vi "Vision Research Phantom Series VI Tree.vi"   [LabVIEW 2013, in "VRI.lvlib"]
doc: "This is the instrument driver for the Dresser DXD Series Precision Digital Pressure Transducer. The VI Tree displays all the user-callable VIs of the instrument driver in an organized table. Look at the \"Getting Started\" VI's to get an idea of how to use this driver in your application."
uses:
  VRI.lvlib
panel:
  # "Vision Research\nPhantom Series\nCamera\nLabVIEW Driver"
  # "SEE DIAGRAM\nFOR VI TREE."
  # "Version 3.0.770.0"
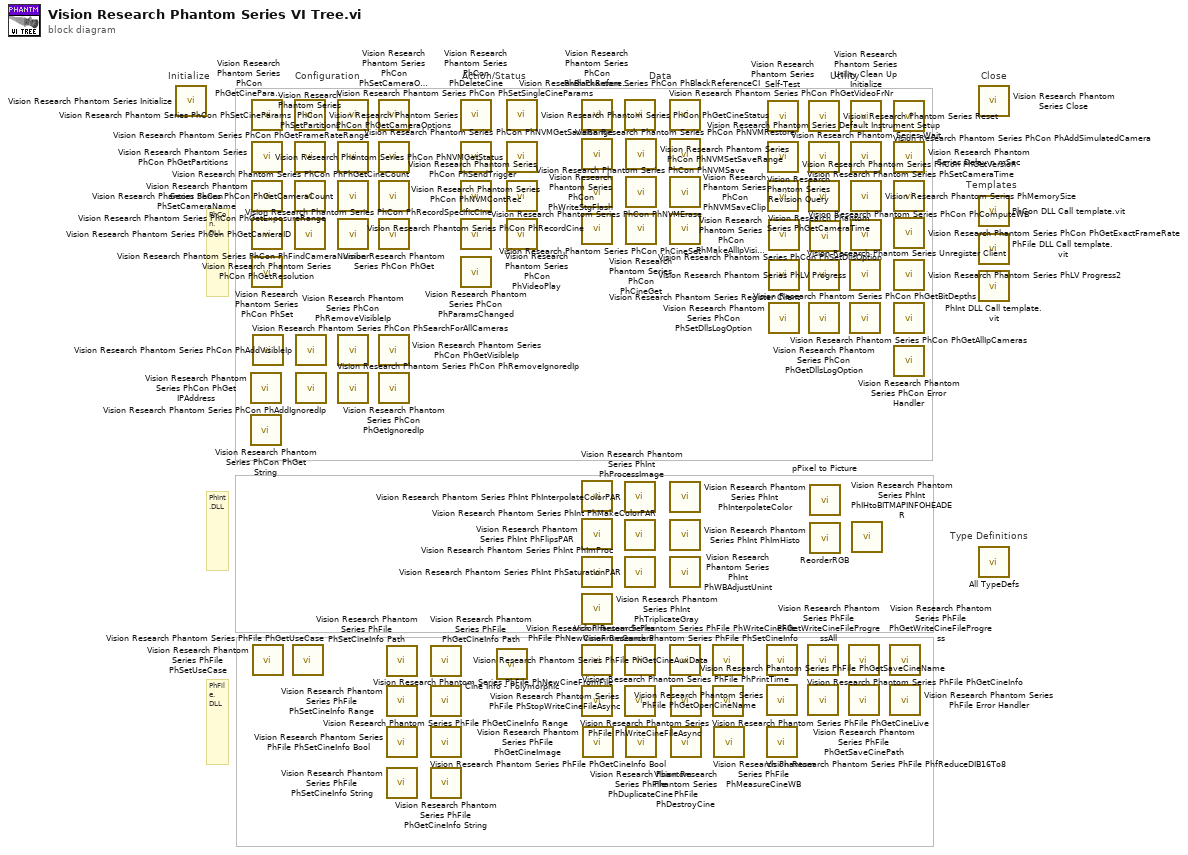
[diagram p0: block diagram]
diagram:
  # "Type Definitions"
  # "PhFile.DLL"
  # "PhInt.DLL"
  # "PhCon.DLL"
  # "Templates"
  # "Configuration"
  # "Utility"
  # "Data"
  # "Action/Status"
  # "Close"
  # "Initialize"
  n1 = call "Vision Research Phantom Series Initialize.vi"() -> ()  [unwired: 5 in, 15 out]
  n2 = call "Vision Research Phantom Series PhCon PhGet IPAddress.vi"() -> ()  [unwired: 17 in, 3 out]
  n3 = call "Vision Research Phantom Series PhCon PhGet String.vi"() -> ()  [unwired: 17 in, 3 out]
  n4 = call "Vision Research Phantom Series PhCon PhGetCineParams.vi"() -> ()  [unwired: 3 in, 17 out]
  n5 = call "Vision Research Phantom Series PhCon PhGetPartitions.vi"() -> ()  [unwired: 3 in, 17 out]
  n6 = call "Vision Research Phantom Series PhCon PhSetCameraName.vi"() -> ()  [unwired: 3 in, 17 out]
  n7 = call "Vision Research Phantom Series PhCon PhGetResolution.vi"() -> ()  [unwired: 4 in, 16 out]
  n8 = call "Vision Research Phantom Series PhCon PhSet.vi"() -> ()  [unwired: 17 in, 3 out]
  n9 = call "Vision Research Phantom Series PhCon PhSearchForAllCameras.vi"() -> ()  [unwired: 2 in, 18 out]
  n10 = call "Vision Research Phantom Series PhFile PhSetUseCase.vi"() -> ()  [unwired: 18 in, 2 out]
  n11 = call "Vision Research Phantom Series PhFile PhGetUseCase.vi"() -> ()  [unwired: 18 in, 2 out]
  n12 = call "Vision Research Phantom Series PhCon PhSetCineParams.vi"() -> ()  [unwired: 4 in, 16 out]
  n13 = call "Vision Research Phantom Series PhCon PhSetPartitions.vi"() -> ()  [unwired: 4 in, 16 out]
  n14 = call "Vision Research Phantom Series PhCon PhGetExposureRange.vi"() -> ()  [unwired: 3 in, 17 out]
  n15 = call "Vision Research Phantom Series PhCon PhGetCameraID.vi"() -> ()  [unwired: 2 in, 18 out]
  n16 = call "Vision Research Phantom Series PhCon PhAddVisibleIp.vi"() -> ()  [unwired: 2 in, 18 out]
  n17 = call "Vision Research Phantom Series PhCon PhAddIgnoredIp.vi"() -> ()  [unwired: 2 in, 18 out]
  n18 = call "Vision Research Phantom Series PhCon PhSetSingleCineParams.vi"() -> ()  [unwired: 3 in, 17 out]
  n19 = call "Vision Research Phantom Series PhCon PhGetFrameRateRange.vi"() -> ()  [unwired: 3 in, 17 out]
  n20 = call "Vision Research Phantom Series PhCon PhGetCameraCount.vi"() -> ()  [unwired: 1 in, 19 out]
  n21 = call "Vision Research Phantom Series PhCon PhFindCameraNumber.vi"() -> ()  [unwired: 2 in, 18 out]
  n22 = call "Vision Research Phantom Series PhCon PhRemoveVisibleIp.vi"() -> ()  [unwired: 2 in, 18 out]
  n23 = call "Vision Research Phantom Series PhCon PhRemoveIgnoredIp.vi"() -> ()  [unwired: 2 in, 18 out]
  n24 = call "Vision Research Phantom Series PhCon PhSetCameraOptions.vi"() -> ()  [unwired: 3 in, 17 out]
  n25 = call "Vision Research Phantom Series PhCon PhGetCameraOptions.vi"() -> ()  [unwired: 2 in, 18 out]
  n26 = call "Vision Research Phantom Series PhCon PhPhGetCineCount.vi"() -> ()  [unwired: 2 in, 18 out]
  n27 = call "Vision Research Phantom Series PhCon PhGet.vi"() -> ()  [unwired: 17 in, 3 out]
  n28 = call "Vision Research Phantom Series PhCon PhGetVisibleIp.vi"() -> ()  [unwired: 1 in, 19 out]
  n29 = call "Vision Research Phantom Series PhCon PhGetIgnoredIp.vi"() -> ()  [unwired: 1 in, 19 out]
  n30 = call "Vision Research Phantom Series PhFile PhSetCineInfo Path.vi"() -> ()  [unwired: 17 in, 3 out]
  n31 = call "Vision Research Phantom Series PhFile PhSetCineInfo Range.vi"() -> ()  [unwired: 17 in, 3 out]
  n32 = call "Vision Research Phantom Series PhFile PhSetCineInfo Bool.vi"() -> ()  [unwired: 17 in, 3 out]
  n33 = call "Vision Research Phantom Series PhFile PhSetCineInfo String.vi"() -> ()  [unwired: 17 in, 3 out]
  n34 = call "Vision Research Phantom Series PhFile PhGetCineInfo Path.vi"() -> ()  [unwired: 17 in, 3 out]
  n35 = call "Vision Research Phantom Series PhFile PhGetCineInfo Range.vi"() -> ()  [unwired: 17 in, 3 out]
  n36 = call "Vision Research Phantom Series PhFile PhGetCineInfo Bool.vi"() -> ()  [unwired: 17 in, 3 out]
  n37 = call "Vision Research Phantom Series PhFile PhGetCineInfo String.vi"() -> ()  [unwired: 17 in, 3 out]
  n38 = call "Vision Research Phantom Series PhCon PhDeleteCine.vi"() -> ()  [unwired: 3 in, 17 out]
  n39 = call "Vision Research Phantom Series PhCon PhNVMContRec.vi"() -> ()  [unwired: 3 in, 17 out]
  n40 = call "Vision Research Phantom Series PhCon PhRecordCine.vi"() -> ()  [unwired: 2 in, 18 out]
  n41 = call "Vision Research Phantom Series PhCon PhRecordSpecificCine.vi"() -> ()  [unwired: 3 in, 17 out]
  n42 = call "Vision Research Phantom Series PhCon PhParamsChanged.vi"() -> ()  [unwired: 2 in, 18 out]
  n43 = call-poly "Cine Info - Polymorphic.vi"() -> ()  [unwired: 17 in, 3 out]
  n44 = call "Vision Research Phantom Series PhCon PhGetCineStatus.vi"() -> ()  [unwired: 3 in, 17 out]
  n45 = call "Vision Research Phantom Series PhCon PhNVMGetStatus.vi"() -> ()  [unwired: 3 in, 17 out]
  n46 = call "Vision Research Phantom Series PhCon PhSendTrigger.vi"() -> ()  [unwired: 2 in, 18 out]
  n47 = call "Vision Research Phantom Series PhCon PhVideoPlay.vi"() -> ()  [unwired: 5 in, 15 out]
  n48 = call "Vision Research Phantom Series PhCon PhBlackReference.vi"() -> ()  [unwired: 3 in, 17 out]
  n49 = call "Vision Research Phantom Series PhCon PhNVMGetSaveRange.vi"() -> ()  [unwired: 2 in, 18 out]
  n50 = call "Vision Research Phantom Series PhCon PhNVMErase.vi"() -> ()  [unwired: 3 in, 17 out]
  n51 = call "Vision Research Phantom Series PhCon PhWriteStgFlash.vi"() -> ()  [unwired: 3 in, 17 out]
  n52 = call "Vision Research Phantom Series PhInt PhProcessImage.vi"() -> ()  [unwired: 17 in, 3 out]
  n53 = call "Vision Research Phantom Series PhInt PhFlipsPAR.vi"() -> ()  [unwired: 4 in, 16 out]
  n54 = call "Vision Research Phantom Series PhInt PhImProc.vi"() -> ()  [unwired: 5 in, 15 out]
  n55 = call "Vision Research Phantom Series PhInt PhTriplicateGray.vi"() -> ()  [unwired: 18 in, 2 out]
  n56 = call "Vision Research Phantom Series PhFile PhNewCineFromFile.vi"() -> ()  [unwired: 2 in, 18 out]
  n57 = call "Vision Research Phantom Series PhFile PhWriteCineFileAsync.vi"() -> ()  [unwired: 17 in, 3 out]
  n58 = call "Vision Research Phantom Series PhFile PhGetCineImage.vi"() -> ()  [unwired: 16 in, 4 out]
  n59 = call "Vision Research Phantom Series PhCon PhBlackReferenceCI.vi"() -> ()  [unwired: 3 in, 17 out]
  n60 = call "Vision Research Phantom Series PhInt PhInterpolateColorPAR.vi"() -> ()  [unwired: 6 in, 14 out]
  n61 = call "Vision Research Phantom Series PhInt PhMakeColorPAR.vi"() -> ()  [unwired: 6 in, 14 out]
  n62 = call "Vision Research Phantom Series PhInt PhSaturationPAR.vi"() -> ()  [unwired: 4 in, 16 out]
  n63 = call "Vision Research Phantom Series PhFile PhNewCineFromCamera.vi"() -> ()  [unwired: 3 in, 17 out]
  n64 = call "Vision Research Phantom Series PhFile PhStopWriteCineFileAsync.vi"() -> ()  [unwired: 19 in, 1 out]
  n65 = call "Vision Research Phantom Series PhCon PhNVMSetSaveRange.vi"() -> ()  [unwired: 3 in, 17 out]
  n66 = call "Vision Research Phantom Series PhCon PhNVMSave.vi"() -> ()  [unwired: 4 in, 16 out]
  n67 = call "Vision Research Phantom Series PhCon PhCineGet.vi"() -> ()  [unwired: 17 in, 3 out]
  n68 = call "Vision Research Phantom Series PhFile PhDuplicateCine.vi"() -> ()  [unwired: 17 in, 3 out]
  n69 = call "Vision Research Phantom Series PhCon PhGetVideoFrNr.vi"() -> ()  [unwired: 2 in, 18 out]
  n70 = call "Vision Research Phantom Series PhCon PhNVMRestore.vi"() -> ()  [unwired: 4 in, 16 out]
  n71 = call "Vision Research Phantom Series PhCon PhNVMSaveClip.vi"() -> ()  [unwired: 6 in, 14 out]
  n72 = call "Vision Research Phantom Series PhCon PhCineSet.vi"() -> ()  [unwired: 17 in, 3 out]
  n73 = call "Vision Research Phantom Series PhInt PhInterpolateColor.vi"() -> ()  [unwired: 5 in, 15 out]
  n74 = call "Vision Research Phantom Series PhInt PhImHisto.vi"() -> ()  [unwired: 5 in, 15 out]
  n75 = call "Vision Research Phantom Series PhInt PhWBAdjustUnint.vi"() -> ()  [unwired: 5 in, 15 out]
  n76 = call "Vision Research Phantom Series PhFile PhWriteCineFile.vi"() -> ()  [unwired: 3 in, 17 out]
  n77 = call "Vision Research Phantom Series PhFile PhPrintTime.vi"() -> ()  [unwired: 18 in, 2 out]
  n78 = call "Vision Research Phantom Series PhFile PhDestroyCine.vi"() -> ()  [unwired: 2 in, 18 out]
  n79 = call "Vision Research Phantom Series PhFile PhGetCineAuxData.vi"() -> ()  [unwired: 5 in, 15 out]
  n80 = call "Vision Research Phantom Series PhFile PhGetCineLive.vi"() -> ()  [unwired: 17 in, 3 out]
  n81 = call "Vision Research Phantom Series PhFile PhMeasureCineWB.vi"() -> ()  [unwired: 5 in, 15 out]
  n82 = call "Vision Research Phantom Series PhFile PhSetCineInfo.vi"() -> ()  [unwired: 17 in, 3 out]
  n83 = call "Vision Research Phantom Series PhFile PhGetOpenCineName.vi"() -> ()  [unwired: 2 in, 18 out]
  n84 = call "Vision Research Phantom Series PhFile PhfReduceDIB16To8.vi"() -> ()  [unwired: 4 in, 16 out]
  n85 = call "Vision Research Phantom Series Self-Test.vi"() -> ()  [unwired: 1 in, 15 out]
  n86 = call "Vision Research Phantom Series Revision Query.vi"() -> ()  [unwired: 1 in, 15 out]
  n87 = call "Vision Research Phantom Series PhGetCameraTime.vi"() -> ()  [unwired: 2 in, 18 out]
  n88 = call "Vision Research Phantom Series PhCon PhMakeAllIpVisible.vi"() -> ()  [unwired: 19 in, 1 out]
  n89 = call "Vision Research Phantom Series Register Client.vi"() -> ()  [unwired: 3 in, 17 out]
  n90 = call "Vision Research Phantom Series PhCon PhSetDllsLogOption.vi"() -> ()  [unwired: 3 in, 17 out]
  n91 = call "Vision Research Phantom Series PhFile PhGetCineInfo.vi"() -> ()  [unwired: 3 in, 17 out]
  n92 = call "Vision Research Phantom Series PhFile PhGetSaveCineName.vi"() -> ()  [unwired: 2 in, 18 out]
  n93 = call "Vision Research Phantom Series Reset.vi"() -> ()  [unwired: 1 in, 15 out]
  n94 = call "Vision Research Phantom Series Default Instrument Setup.vi"() -> ()  [unwired: 1 in, 15 out]
  n95 = call "Vision Research Phantom Series PhSetCameraTime.vi"() -> ()  [unwired: 2 in, 18 out]
  n96 = call "Vision Research Phantom Series Unregister Client.vi"() -> ()  [unwired: 1 in, 19 out]
  n97 = call "Vision Research Phantom Series PhCon PhGetDllsLogOption.vi"() -> ()  [unwired: 2 in, 18 out]
  n98 = call "Vision Research Phantom Series PhCon PhComputeWB.vi"() -> ()  [unwired: 6 in, 14 out]
  n99 = call "pPixel to Picture.vi"() -> ()  [unwired: 3 in, 1 out]
  n100 = call "ReorderRGB.vi"() -> ()  [unwired: 1 in, 1 out]
  n101 = call "Vision Research Phantom Series PhFile PhGetWriteCineFileProgressAll.vi"() -> ()  [unwired: 17 in, 3 out]
  n102 = call "Vision Research Phantom Series PhFile PhGetSaveCinePath.vi"() -> ()  [unwired: 2 in, 18 out]
  n103 = call "Vision Research Phantom Series PhLV Progress.vi"() -> ()  [unwired: 3 in, 17 out]
  n104 = call "Vision Research Phantom Series PhCon PhGetBitDepths.vi"() -> ()  [unwired: 2 in, 18 out]
  n105 = call "Vision Research Phantom Series Utility Clean Up Initialize.vi"() -> ()  [unwired: 1 in, 15 out]
  n106 = call "Vision Research Phantom Series Wait.vi"() -> ()  [unwired: 1 in, 15 out]
  n107 = call "Vision Research Phantom Series PhMemorySize.vi"() -> ()  [unwired: 2 in, 18 out]
  n108 = call "Vision Research Phantom Series PhCon PhSetDllsOption.vi"() -> ()  [unwired: 18 in, 2 out]
  n109 = call "Vision Research Phantom Series PhInt PhIHtoBITMAPINFOHEADER.vi"() -> ()  [unwired: 18 in, 2 out]
  n110 = call "Vision Research Phantom Series PhFile PhGetWriteCineFileProgress.vi"() -> ()  [unwired: 17 in, 3 out]
  n111 = call "Vision Research Phantom Series PhFile Error Handler.vi"() -> ()  [unwired: 2 in, 18 out]
  n112 = call "Vision Research Phantom Series PhCon PhAddSimulatedCamera.vi"() -> ()  [unwired: 3 in, 17 out]
  n113 = call "Vision Research Phantom Series Delay n mSec.vi"() -> ()  [unwired: 2 in, 14 out]
  n114 = call "Vision Research Phantom Series PhCon PhGetVersion.vi"() -> ()  [unwired: 3 in, 17 out]
  n115 = call "Vision Research Phantom Series PhCon PhGetExactFrameRate.vi"() -> ()  [unwired: 4 in, 16 out]
  n116 = call "Vision Research Phantom Series PhLV Progress2.vi"() -> ()  [unwired: 4 in, 16 out]
  n117 = call "Vision Research Phantom Series PhCon PhGetAllIpCameras.vi"() -> ()  [unwired: 17 in, 3 out]
  n118 = call "Vision Research Phantom Series PhCon Error Handler.vi"() -> ()  [unwired: 2 in, 18 out]
  n119 = call "Vision Research Phantom Series Close.vi"() -> ()  [unwired: 1 in, 19 out]
  n120 = call "PhCon DLL Call template.vit"() -> ()  [unwired: 2 in, 18 out]
  n121 = call "PhFile DLL Call template.vit"() -> ()  [unwired: 2 in, 18 out]
  n122 = call "PhInt DLL Call template.vit"() -> ()  [unwired: 2 in, 18 out]
  n123 = call "All TypeDefs.vi"() -> ()  [unwired: 1 out]
